vi "GetValue.vi"(8 "error in":errorcluster, 11 "UnsignedByte in":refnum<class "UnsignedByte.lvclass">) -> (0 "error out":errorcluster, 2 "Value":u8, 3 "UnsignedByte out":refnum<class "UnsignedByte.lvclass">)   [LabVIEW 2021, in "ProligentXMLGenerator.lvlib" / "UnsignedByte.lvclass"]
uses:
  UnsignedByte.lvclass
  UnsignedByte.lvclass/UnsignedByte.ctl
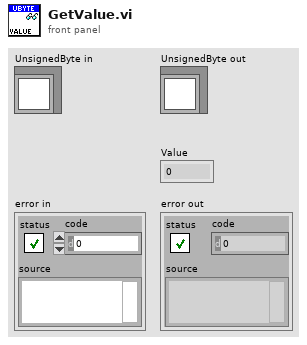
[diagram p1: front panel]
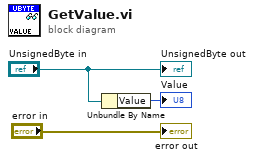
[diagram p0: block diagram]
diagram:
  n1 = Unbundle By Name("UnsignedByte in") -> ("Value"=→"Value":u8)
  "error out" <- "error in"
  "UnsignedByte out" <- "UnsignedByte in"
